vi "set_wavelength.vi"(8 "error in (no error)":errorcluster, 10 "Spectrometer Handle":u32, 11 "wavelength":dbl) -> (0 "error out":errorcluster, 2 "Spectrometer handle":u32, 3 "Filter Number":dbl=5.0)   [LabVIEW 2018]
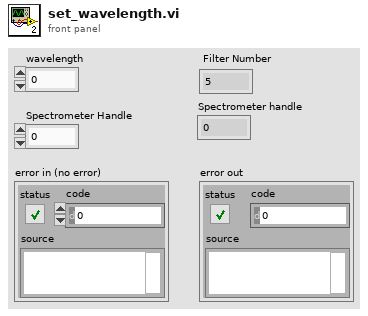
[diagram p1: front panel]
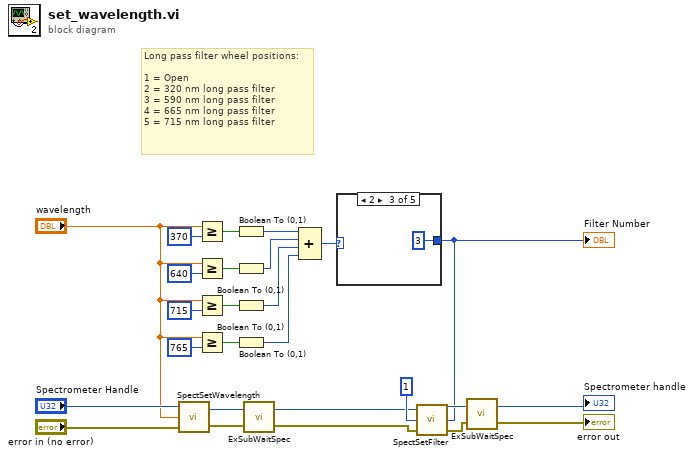
[diagram p0: block diagram]
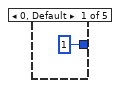
[diagram p2: hidden frame]
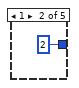
[diagram p3: hidden frame]
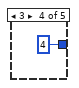
[diagram p4: hidden frame]
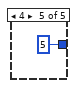
[diagram p5: hidden frame]
diagram:
  # "Long pass filter wheel positions:\n\n1 = Open\n2 = 320 nm long pass filter\n3 = 590 nm long pass filter\n4 = 665 nm long pass filter\n5 = 715 nm long pass filter"
  n1 = call "SpectSetWavelength.vi"("error in"="error in (no error)", "Wavelength"="wavelength", "Spectrometer Handle"="Spectrometer Handle") -> ("error out"=w23:errorcluster, "Spectrumeter Handle"=w16:u32)
  n2 = Greater Or Equal?(x="wavelength", y=370) -> (x >= y?=w11:bool)
  n3 = Greater Or Equal?(x="wavelength", y=640) -> (x >= y?=w10:bool)
  n4 = Greater Or Equal?(x="wavelength", y=715) -> (x >= y?=w9:bool)
  n5 = Greater Or Equal?(x="wavelength", y=765) -> (x >= y?=w8:bool)
  n6 = Boolean To (0,1)(Boolean=w11) -> (0, 1=w7:i16)
  n7 = Boolean To (0,1)(Boolean=w10) -> (0, 1=w6:i16)
  n8 = Boolean To (0,1)(Boolean=w9) -> (0, 1=w5:i16)
  n9 = Boolean To (0,1)(Boolean=w8) -> (0, 1=w4:i16)
  n10 = call "ExSubWaitSpec.vi"("error in (no error)"=w23, "Spectrometer Handle"=w16) -> ("error out"=w19:errorcluster, "Spectrometer handle"=w18:u32)
  n11 = Compound Arithmetic op=ADD(w7, w6, w5, w4) -> (w3:i16)
  n12 = case shown="2" w3 {
    tunnel: [1 2 3 4 5] -> w2
    frame 0, Default {
    }
    frame 1 {
    }
    frame 2 {
    }
    frame 3 {
    }
    frame 4 {
    }
  }
  "Filter Number" <- w2
  n13 = call "SpectSetFilter.vi"("Filter Number"=w2, "error in"=w19, "Filter Wheel Number"=1, "Spectrometer Handle"=w18) -> ("error out"=w21:errorcluster, "Spectrometer Handle"=w20:u32)
  n14 = call "ExSubWaitSpec.vi"("error in (no error)"=w21, "Spectrometer Handle"=w20) -> ("error out"=→"error out":errorcluster, "Spectrometer handle"=→"Spectrometer handle":u32)
